vi "Main.vi"(8 "Error In":errorcluster) -> (0 "Error Out":errorcluster)   [LabVIEW 2017, in "Auto cycle.lvlib"]
uses:
  Auto cycle.lvlib
  System Control/Main controller.lvlib
  Events/Events.lvlib
  Controls/Commands [enum].ctl
  System Control/CTLs/Test indicators.ctl
  Test params.ctl
  Scope/Scope.lvlib
  System Control/CTLs/Test Controls.ctl
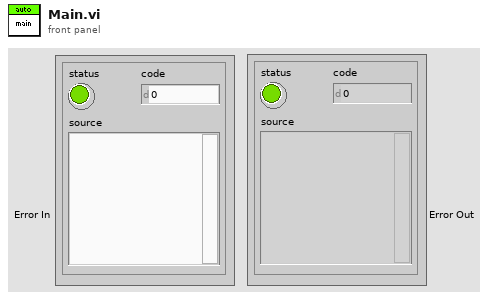
[diagram p1: front panel]
types:
  T1 = typedef "Test params.ctl" = cluster{"Config":T2, "Indicators":T3}
  T2 = typedef "Main controller.lvlib/Test Controls.ctl" = cluster{"Amplification Factor":dbl, "100% reflectance standard":dbl, "Calculation Method":enum16{"Reflectance", "Transmission", "Kubelka-Munk"}, "Option to discard new data?":bool, "Mode":enum32{"Spectrum", "Kinetic"}, "Number of averages":u32}
  T3 = typedef "Main controller.lvlib/Test indicators.ctl" = cluster{"DAQ Background Level (V)":dbl, "A-Test Counter":i32, "B-test counter":i32, "Type":enum32{"A-test", "B-test"}, "Scope Background Level (Amps)":dbl, "TAS only?":bool}
  T4 = typedef "Events.lvlib/Refs [cluster].ctl" = cluster{"Exit":refnum<user-event>, "Controller":refnum<user-event>, "System Error":refnum<user-event>, "UI":refnum<user-event>, "Example Module":refnum<user-event>, "Shutter":refnum<user-event>, "Monochromator":refnum<user-event>, "DAQ":refnum<user-event>, "Scope":refnum<user-event>, "Auto cycle":refnum<user-event>, "Processing":refnum<user-event>, "File IO":refnum<user-event>, "Colour wheel":refnum<user-event>}
  T5 = typedef "Auto cycle.lvlib/Commands [enum].ctl" = enum16{"Start", "Stop", "Send config", "Run test", "Post-processing"}
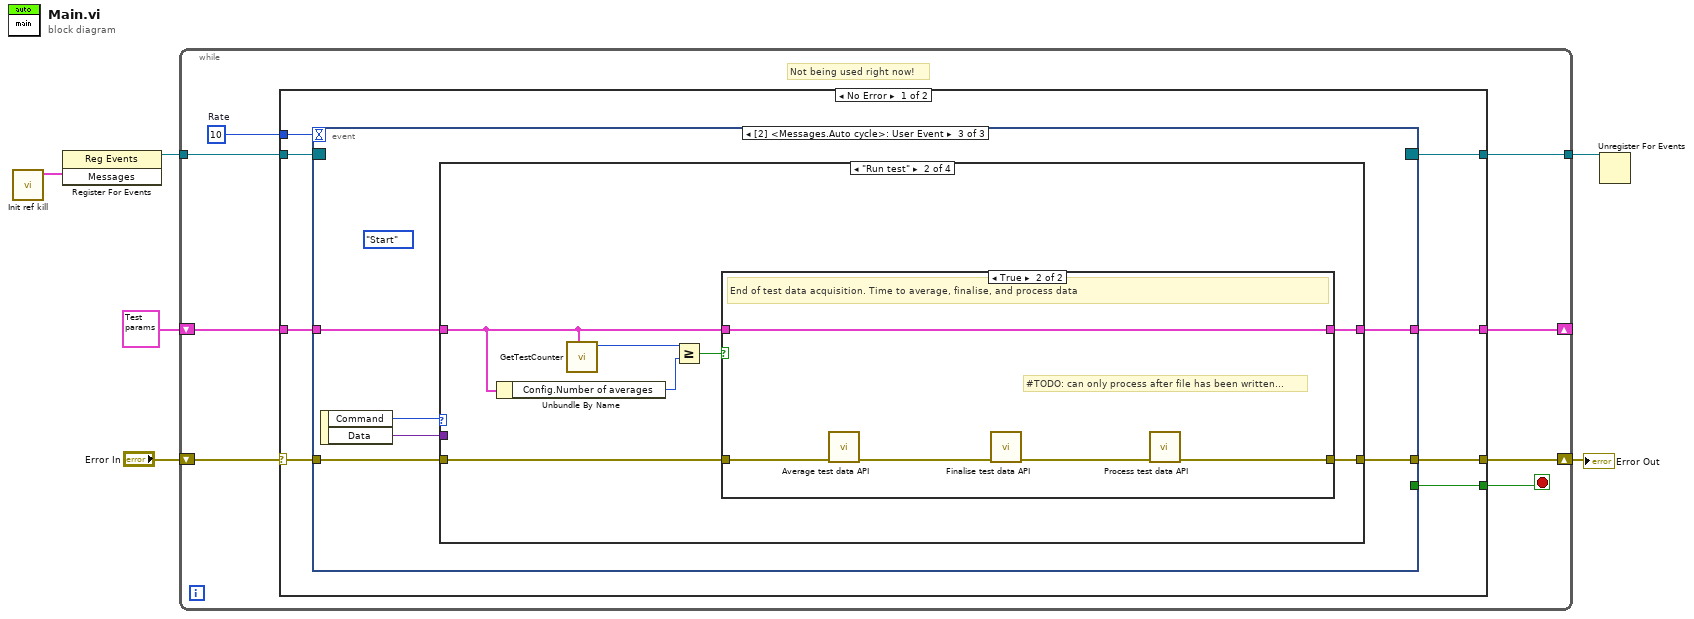
[diagram p0: block diagram]
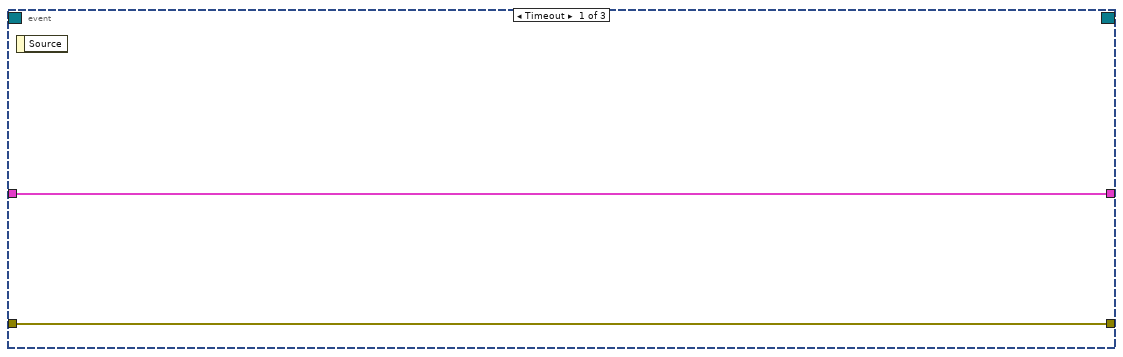
[diagram p2: hidden frame]
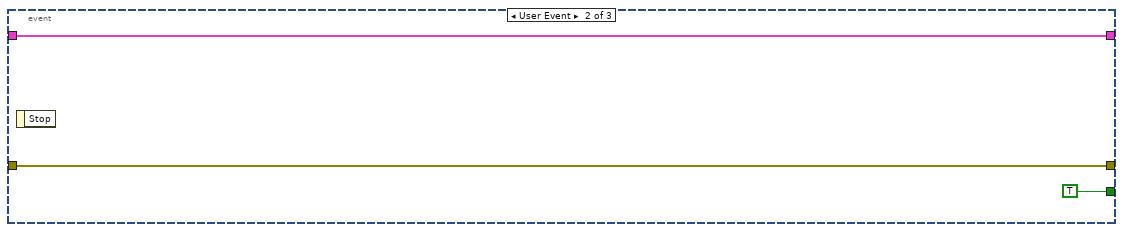
[diagram p3: hidden frame]
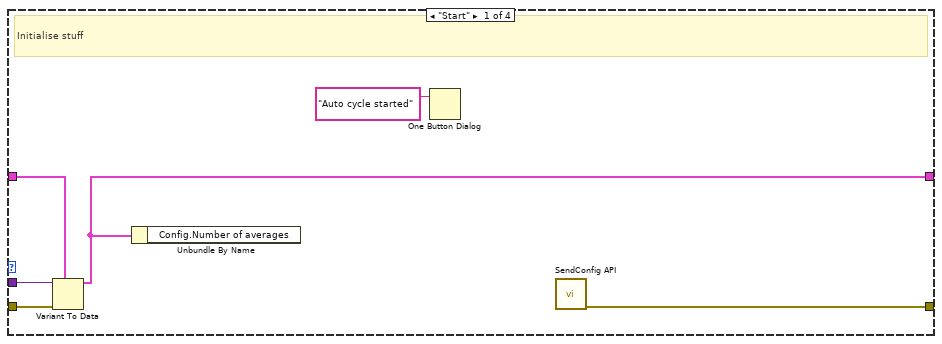
[diagram p4: hidden frame]
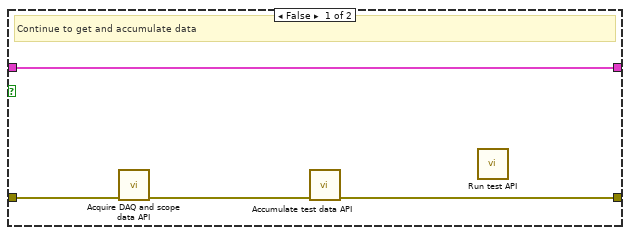
[diagram p5: hidden frame]
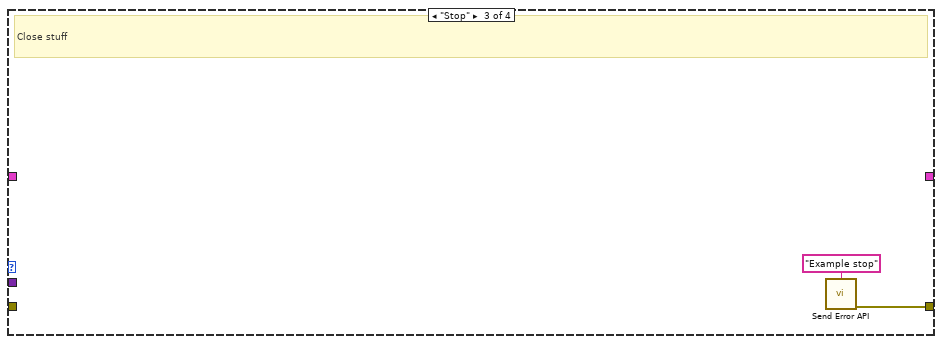
[diagram p6: hidden frame]
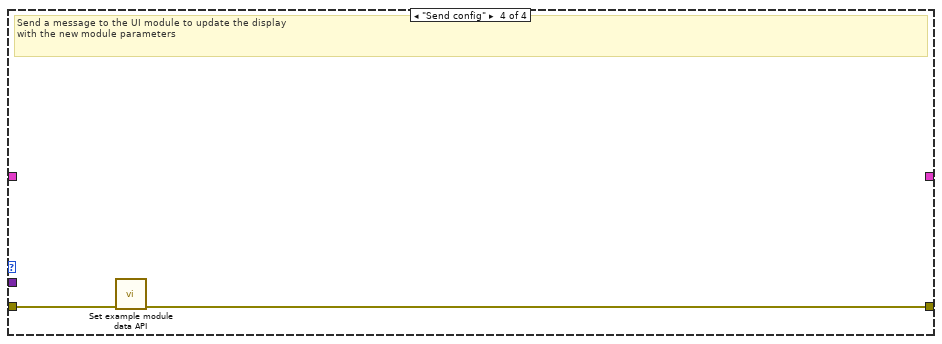
[diagram p7: hidden frame]
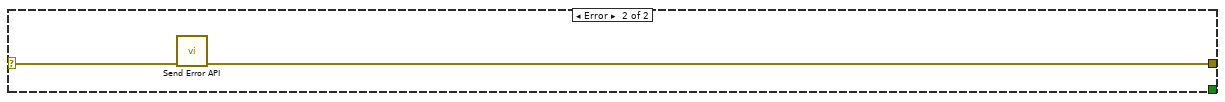
[diagram p8: hidden frame]
diagram:
  n1 = call "Init ref kill.vi"() -> ("Messages"=w6:T4)  [unwired: 10 in, 1 out]
  n2 = register-events(w6) -> (reference out=w5:refnum<event-registration>)  [unwired: 2 in, 1 out]
  n3 = while {
    tunnel: w5 -> [w14]
    tunnel: [w11] -> w4
    shift-right: [w8] -> w2
    shift-left: "Error In" -> [w7]
    shift-right: [w9] -> _
    shift-left: T1 {"Config"={"Amplification Factor"=2.0, "100% reflectance standard"=2.0, "Calculation Method"=enum."Reflectance", "Option to discard new data?"=FALSE, "Mode"=enum."Spectrum", "Number of averages"=0}, "Indicators"={"DAQ Background Level (V)"=2.0, "A-Test Counter"=2, "B-test counter"=2, "Type"=enum."A-test", "Scope Background Level (Amps)"=2.0, "TAS only?"=FALSE}} ("Test") -> [w10]
    stop <- w12 stop-if-true
    w13 = 10  # Rate
    # "Not being used right now!"
    n4 = case shown="No Error" w7 {
      selector: w7 -> [w15 w61]
      tunnel: w14 -> [w22 _]
      tunnel: w13 -> [w21 _]
      tunnel: [w20 _] -> w12
      tunnel: [w19 _] -> w11
      tunnel: w10 -> [w18 _]
      tunnel: [w17 _] -> w9
      tunnel: [w16 w60] -> w8
      frame No Error {
        n5 = event shown="[2] <Messages.Auto cycle>: User Event" {
          selector: w22 -> [_ _ _]
          dyn-events: [_ _ _] -> w19
          timeout: w21 -> [_ _ _]
          tunnel: [_ TRUE _] -> w20
          tunnel: w15 -> [w23 w25 w31]
          tunnel: [w23 w25 w30] -> w16
          tunnel: w18 -> [w24 w26 w29]
          tunnel: [w24 w26 w28] -> w17
          event Timeout {
            n6 = event-data() -> ()  [unwired: 1 in, 1 out]
          }
          event User Event {
            n7 = event-data() -> ()  [unwired: 1 in, 1 out]
          }
          event User Event {
            (unwired) Commands_[enum]."Start" ("Enum")
            n8 = event-data() -> ("Command"=w33:T5, "Data"=w32:variant)  [unwired: 1 in]
            n9 = case shown="\"Run test\"" w33 {
              tunnel: w32 -> [w36 _ _ _]
              tunnel: w31 -> [w37 w40 _ w59]
              tunnel: [w38 w41 w57 w58] -> w30
              tunnel: w29 -> [w35 w42 _ _]
              tunnel: [w34 w43 _ _] -> w28
              frame "Start" {
                # "Initialise stuff"
                n10 = Variant To Data(error in=w37, type=w35, Variant=w36) -> (data=w34:T1)  [unwired: 1 out]
                n11 = Unbundle By Name(w34) -> ()  [unwired: 1 out]
                n12 = One Button Dialog(message="Auto cycle started") -> ()  [unwired: 1 in, 1 out]
                n13 = call "SendConfig API.vi"() -> ("Error Out"=w38:errorcluster)  [unwired: 11 in]
              }
              frame "Run test" {
                n14 = Unbundle By Name(w42) -> ("Config.Number of averages"=w45:u32)
                n15 = call "GetTestCounter.vi"("Test"=w42) -> ("Current test counter"=w46:i32)  [unwired: 10 in]
                n16 = Greater Or Equal?(x=w46, y=w45) -> (x >= y?=w44:bool)
                n17 = case shown="True" w44 {
                  tunnel: [w47 w53] -> w43
                  tunnel: w42 -> [w47 w53]
                  tunnel: [w48 w52] -> w41
                  tunnel: w40 -> [w49 w51]
                  frame False {
                    # "Continue to get and accumulate data"
                    n18 = call "Acquire DAQ and scope data API.vi"("Error In"=w49) -> ("Error Out"=w50:errorcluster)  [unwired: 10 in]
                    n19 = call "Accumulate test data API.vi"("Error In"=w50) -> ("Error Out"=w48:errorcluster)  [unwired: 10 in]
                    n20 = call "Run test API.vi"() -> ()  [unwired: 11 in, 1 out]
                  }
                  frame True {
                    # "#TODO: can only process after file has been written..."
                    # "End of test data acquisition. Time to average, finalise, and process data"
                    n21 = call "Average test data API.vi"("Error In"=w51) -> ("Error Out"=w55:errorcluster)  [unwired: 10 in]
                    n22 = call "Finalise test data API.vi"("Error In"=w55) -> ("Error Out"=w54:errorcluster)  [unwired: 10 in]
                    n23 = call "Process test data API.vi"("Error In"=w54) -> ("Error Out"=w52:errorcluster)  [unwired: 10 in]
                  }
                }
              }
              frame "Stop" {
                # "Close stuff"
                n24 = call "Send Error API.vi"("Error"="Example stop") -> ("Error Out"=w57:errorcluster)  [unwired: 10 in]
              }
              frame "Send config" {
                # "Send a message to the UI module to update the display \nwith the new module parameters"
                n25 = call "Set example module data API.vi"("Error In"=w59) -> ("Error Out"=w58:errorcluster)  [unwired: 10 in]
              }
            }
          }
        }
      }
      frame Error {
        n26 = call "Send Error API.vi"("Error Cluster"=w61) -> ("Error Out"=w60:errorcluster)  [unwired: 10 in]
      }
    }
  }
  "Error Out" <- w2
  n27 = Unregister For Events(event registration refnum=w4) -> ()  [unwired: 1 in, 1 out]
